vi "NodeUI.vi"() -> ()   [LabVIEW 2013, in "NISE_CEF_Node.lvclass"]
doc: "UI that will be called when the node is selected."
uses:
  NISE_CEF_Node.lvclass
  NodeRef.ctl
  <vilib>/NI/AMC/Message Queue.ctl
  <vilib>/NI/AMC/Message.ctl
  <vilib>/NI/Tools/Keyed Array/KeyedArray.ctl
  UserEventRef.ctl
  Controls/EventCluster.ctl
  <vilib>/NI/AMC/Create Single Message.vi
  <vilib>/NI/AMC/Update Message Routing Info.vi
  <vilib>/NI/AMC/Send Message.vi
  <vilib>/NI/AMC/AMC.lvlib
  <vilib>/NI/Tools/Keyed Array/Tools_KeyedArray.lvlib
  NISE_CEF_TreeControl.lvlib
panel:
  out "Numeric":i32
  in  "user event":T1
  in  "main queue":T2
  in  "String":string
  in  "node ref":T3
  # "Default node UI\nNo UI has been created for this type of node."
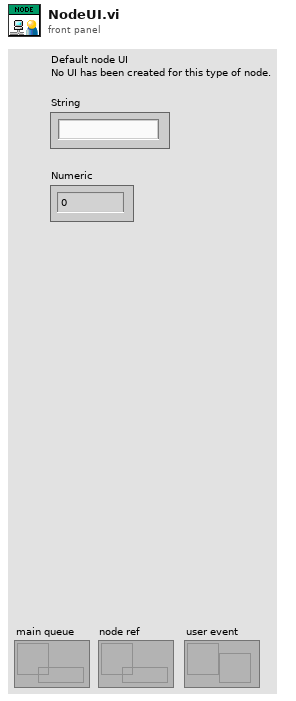
[diagram p1: front panel]
types:
  T1 = typedef "NISE_CEF_Node.lvclass/UserEventRef.ctl" = refnum<user-event>
  T2 = typedef "AMC.lvlib/Message Queue.ctl" = refnum<queue>
  T3 = typedef "NISE_CEF_Node.lvclass/NodeRef.ctl" = refnum<data-value>
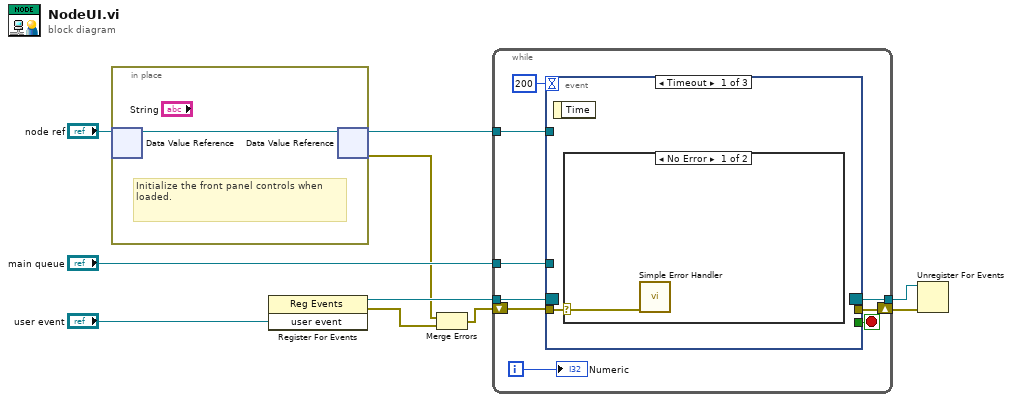
[diagram p0: block diagram]
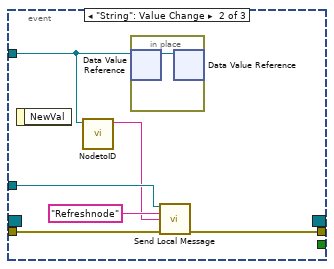
[diagram p3: hidden frame]
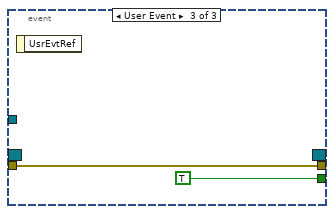
[diagram p4: hidden frame]
diagram:
  n1 = in-place {
    # "Initialize the front panel controls when loaded."
    n2 = in-place-dvr #1("node ref") -> (w11:refnum<class "NISE_CEF_Node.lvclass">)  [unwired: 1 out]
    n3 = in-place-dvr #1(w11) -> (w9:T3, w3:errorcluster)
  }
  n4 = register-events("user event") -> (reference out=w6:refnum<event-registration>, error out=w2:errorcluster)  [unwired: 2 in]
  n5 = Merge Errors(w3, w2) -> (w1:errorcluster)
  n6 = while {
    tunnel: w9 -> [w20]
    tunnel: "main queue" -> [w19]
    tunnel: w6 -> [w17]
    tunnel: [w16] -> w5
    shift-right: [w14] -> w4
    shift-left: w1 -> [w13]
    i -> [w12]
    stop <- w15 stop-if-true
    n7 = event shown="[0] Timeout" {
      selector: w17 -> [_ _ _]
      dyn-events: [_ _ _] -> w16
      timeout: 200 -> [_ _ _]
      tunnel: w20 -> [_ w26 _]
      tunnel: w19 -> [_ w27 _]
      tunnel: [_ _ TRUE] -> w15
      tunnel: [_ w24 w30] -> w14
      tunnel: w13 -> [w21 w23 w30]
      event Timeout {
        n8 = event-data() -> ()  [unwired: 1 in, 1 out]
        n9 = case shown="No Error" w21 {
          selector: w21 -> [w22 _]
          frame No Error {
            n10 = call <vilib>:"Simple Error Handler.vi"("error in (no error)"=w22) -> ()  [unwired: 4 in, 5 out]
          }
          frame Error {
          }
        }
      }
      event "String": Value Change {
        n11 = event-data() -> ()  [unwired: 1 in, 1 out]
        n12 = call "NodetoID.vi"("node ref"=w26) -> ("ID"=w25:string)  [unwired: 9 in, 1 out]
        n13 = in-place {
          n14 = in-place-dvr #2(w26) -> (w29:refnum<class "NISE_CEF_Node.lvclass">)  [unwired: 1 out]
          n15 = in-place-dvr #2(w29) -> ()  [unwired: 2 out]
        }
        n16 = call <vilib>:"Send Local Message.vi"("message queue in"=w27, "message name"="Refreshnode" ("Message Name"), "message value"=w25, "error in"=w23) -> ("error out"=w24:errorcluster)  [unwired: 9 in, 2 out]
      }
      event User Event {
        n17 = event-data() -> ()  [unwired: 1 in, 1 out]
      }
    }
    "Numeric" <- w12
  }
  n18 = Unregister For Events(event registration refnum=w5, error in=w4) -> ()  [unwired: 1 out]
